vi "Dashboard Main.vi"() -> ()   [LabVIEW 2017]
uses:
  <vilib>/Utility/miscctls.llb/LVRowAndColumnTypeDef.ctl
  <vilib>/event_ctls.llb/eventvkey.ctl
  <vilib>/Rock Robotics/Network Tables/NT Read Numeric Array.vi
  <vilib>/Rock Robotics/Network Tables/NT Read Boolean.vi
  <vilib>/Rock Robotics/Network Tables/NT Write Boolean.vi
  <vilib>/Rock Robotics/WPI/Dashboard/WPI_DashboardLogging Global.vi
panel:
  in  "Camera Settings Right":T1={"Frame Rate"=30, "Compression"=30, "Size"=1, "DB Camera Config"=FALSE} {"Frame Rate" scale=1.0..30.0; "Compression" scale=100.0..-1.0; "Size" items=["640x480", "320x240", "160x120"]}
  in  "Camera Name Right":string(combo)="No Camera Selection"
  out "Camera Info":cluster{"Mbps LED":bool, "Mbps":dbl, "fps":dbl} {"fps" format="%#.1g"; "Mbps" format="%#.1g"}
  in  "Camera Settings":T1={"Frame Rate"=30, "Compression"=30, "Size"=1, "DB Camera Config"=FALSE} {"Frame Rate" scale=1.0..30.0; "Compression" scale=100.0..-1.0; "Size" items=["640x480", "320x240", "160x120"]}
  in  "TCP":refnum<k5>
  in  "Rec Mode":enum32{"Stop", "Record", "Playback"}(radio)
  out "Robot IP":string
  out "Image Message":string="Timeout in Camera Communications"
  in  "Dashboard Tab":T2(tab)
  in  "Select Auto":string(combo)="Select Autonomous ..."
  out "NT Connection":bool
  out "MotorChart R":cluster{"Numeric":dbl, "Numeric":dbl}(graph)
  out "MotorChart L":cluster{"Numeric":dbl, "Numeric":dbl}(graph)
  out "MotorSliders R":cluster{"MotorSlide1":dbl, "MotorSlide2":dbl} {"MotorSlide2" scale=-1.0..1.0 scale format="%#_2e"; "MotorSlide1" scale=-1.0..1.0 scale format="%#_2e"}
  out "MotorSliders L":cluster{"MotorSlide1":dbl, "MotorSlide2":dbl} {"MotorSlide2" scale=-1.0..1.0 scale format="%#_2e"; "MotorSlide1" scale=-1.0..1.0 scale format="%#_2e"}
  out "JS1 Z":dbl(slide) scale=-1.0..1.0 scale format="%#_2e"
  out "JS1 Graph":cluster{"X":dbl, "Y":dbl}[](graph)
  out "JS1 Buttons":T3
  out "JS2 Z":dbl(slide) scale=-1.0..1.0 scale format="%#_2e"
  out "JS2 Graph":cluster{"X":dbl, "Y":dbl}[](graph)
  out "JS2 Buttons":T3
  out "Mode":T4(ring)=enum."Auto Disabled"
  out "Camera Image Right":T5(plugin-control)
  in  "Go Fast":bool
  in  "Trim":dbl(slide) scale=0.0..1.0
  in  "Forward?":bool
  in  "If you want to go straight, how far?":dbl
  in  "How fast do you want it to go?":dbl
  in  "If you want to deliver a cube, where?":string(combo)
  in  "Which Auto Program do you want?":string(combo)
  out "Upper lift limit":bool
  out "lower lift limit":bool
  out "gyro":dbl(knob) scale=0.0..360.0
  out "Gauge":dbl(knob) scale=0.0..90.0
  in  "Clear Sticky Faults":bool
  in  "Intake Angle Speed":dbl
  out "Intake angle encoder":dbl
  out "NavX Pitch":dbl
  out "Right encoder":dbl
  out "Pigeon Pitch":dbl
  out "left encoder":dbl
  in  "Test Slider":dbl(slide) scale=0.0..100.0 scale format="%#_3g"
  in  "On/Off":bool caption="Solenoid"
  in  "Test Name":u16(ring) items=["Select the test to run..."]
  in  "Test Tree":string(tree)
  in  "Motor":cluster{"Value":dbl, "Enable":bool} {"Value" scale=-1.0..1.0 scale format="%#_3g"}
  out "Progress":T6 {"Test Progress" scale=0.0..100.0}
  in  "Rev/Fwd":cluster{"Forward":bool, "Reverse":bool}
  in  "Test Ring":u16(ring) items=["Monochrome", "Color"]
  out "Cmd Status":string
  in  "Execute Command":bool
  in  "Command Params":string[][](table)
  in  "Command Selection":i32(listbox)
  in  "CheckList":i32(listbox)
  out "Tree":string(tree)
  out "Camera Image":T5(plugin-control)
  out "Background":bool
  in  "Camera Name":string(combo)="No Camera Selection"
  # "HW"
  # "HW"
  # "Joysticks"
  # "Drive Motors"
  # "Front"
  # "Right"
  # "Left"
  # "Back"
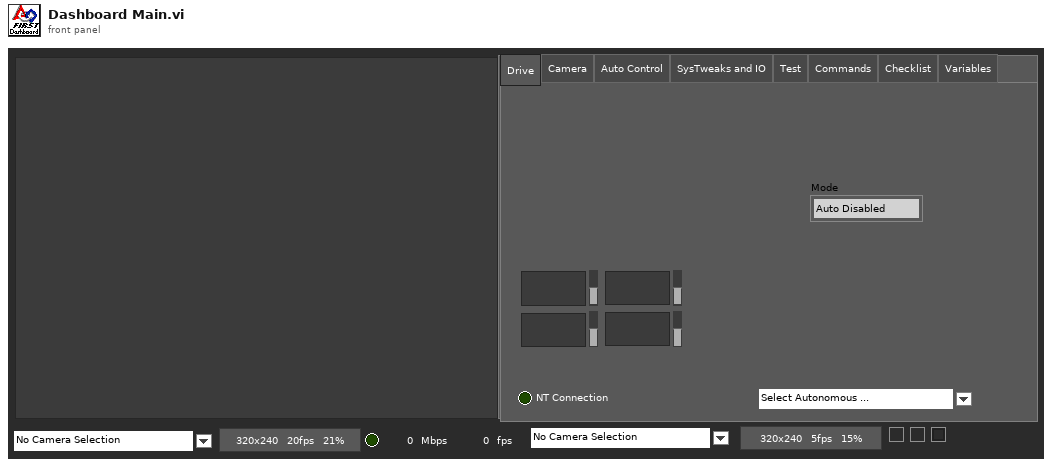
[diagram p1: front panel]
types:
  T1 = cluster{"Frame Rate":i32, "Compression":i32, "Size":u16, "DB Camera Config":bool}
  T2 = enum32{"Drive", "Camera", "Auto Control", "SysTweaks and IO", "Test", "Commands", "Checklist", "Variables"}
  T3 = cluster{bool, bool, bool, bool, bool, bool, bool, bool, bool, bool, bool, bool}
  T4 = enum8{"Tele-Op Disabled", "Tele-Op Enabled", "Auto Disabled", "Auto Enabled", "Test Disabled", "Test Enabled", "Disconnected", "No Code", "E-Stop"}
  T5 = typedef "IMAQ Image.ctl" = refnum<image>
  T6 = cluster{"Test Progress":u8, "Test Progress Text":string}
  T7 = cluster{"Save Path":path, "Interval (s)":dbl, "Keep":i32}
  T8 = enum32{"Drive", "Camera", "Basic", "Custom", "Test", "Commands", "Checklist", "Variables"}
  T9 = typedef "Image Type" = u32
  T10 = cluster{"IDs":cluster{"RPC field ID":u16, "Unique ID":u16}, "String":string}
  T11 = cluster{"Error Strings":string, "Disable Counts":cluster{u16, u16}, "Rail Faults":cluster{u16, u16, u16}, "Robot IP":string, "DB Mode":u8, "Event Info":cluster{"Name":string, "Type":u8, "Number":u16, "Replay":u8}}
  T12 = cluster{"Storage":cluster{"Disk Free":u64, "RAM Block":u32, "RAM free":u32}, "CPU Utilization":cluster{"CPU % ISR":sgl, "CPU % Time Crit":sgl, "CPU % Timed Str":sgl, "CPU % High":sgl, "CPU % Above":sgl, "CPU % Normal":sgl, "CPU % Low":sgl}, "CAN":cluster{"% Bus Utilization":sgl, "Bus Off Cnt":u32, "TX_FIFO Full Cnt":u32, "Receive Error Cnt":u8, "Transmit Error Cnt":u8}, "HID":cluster{"HID Outputs":u32, "Rumble Low":u16, "Rumble High":u16}[]}
  T13 = cluster{"Status bits":cluster{"Test Mode":bool, "Autonomous":bool, "Enabled":bool, "Code Start":bool, "Brownout":bool, "Reserved 2":bool, "Reserved 3":bool, "E-Stop":bool}, "Code Trace":cluster{"Disabled":bool, "TeleOp":bool, "Auto":bool, "Test":bool}, "Controller Type":enum16{"unknown", "cRIO", "roboRio"}, "Code?":enum16{"unknown", "noCode", "code"}, "Battery V":dbl}
  T14 = cluster{"Control Bits":cluster{"TestMode":bool, "Autonomous":bool, "Enabled":bool, "FMS Present":bool, bool, bool, bool, "E-Stop":bool}, "Team Station ":u8, "Countdown":sgl, "Joystick Values":cluster{"Axes":dbl[], "Buttons":bool[], "POVs":i16[]}[]}
  T15 = cluster{"Axes":dbl[], "Buttons":bool[], "POVs":i16[]}[]
  T16 = cluster{"Numeric Array[0]":dbl, "Numeric Array[1]":dbl, "Numeric Array[2]":dbl, "Numeric Array[3]":dbl, "Numeric Array[4]":dbl, "Numeric Array[5]":dbl, "Numeric Array[6]":dbl, "Numeric Array[7]":dbl, "Numeric Array[8]":dbl}
  T17 = cluster{"Axes":dbl[], "Buttons":bool[], "POVs":i16[]}
  T18 = cluster{"Buttons[0]":bool, "Buttons[1]":bool, "Buttons[2]":bool, "Buttons[3]":bool, "Buttons[4]":bool, "Buttons[5]":bool, "Buttons[6]":bool, "Buttons[7]":bool, "Buttons[8]":bool, "Buttons[9]":bool, "Buttons[10]":bool, "Buttons[11]":bool}
  T19 = cluster{"Camera Image":refnum<vi>, "Dashboard Tab":refnum<vi>, "Background":refnum<vi>, "Rec Mode":refnum<vi>, "Test Slider":refnum<vi>, "On/Off ":refnum<vi>, "Test Ring":refnum<vi>, "Rev/Fwd":refnum<vi>, "Test Name":refnum<vi>, "Motor":refnum<vi>, "Progress":refnum<vi>, "CheckList":refnum<vi>, "Tree":refnum<vi>, "Test Tree":refnum<vi>, "Command Params":refnum<vi>, "Command Selection":refnum<vi>, "Execute Command":refnum<vi>, "Cmd Status":refnum<vi>, "Camera Settings":refnum<vi>, "Camera Name":refnum<vi>, "Camera Info":refnum<vi>, "Camera Settings Right":refnum<vi>, "Camera Name Right":refnum<vi>, "Camera Image Right":refnum<vi>}
  T20 = cluster{"Camera Name Right":string, string, "Saved DB Images Info":cluster{"Save Path":path, "Interval (s)":dbl, "Keep":i32}}
  T21 = cluster{"Camera Name":string, string, "Saved DB Images Info":cluster{"Save Path":path, "Interval (s)":dbl, "Keep":i32}}
  T22 = cluster{"Operation":enum16{"Update", "Clear"}, "Color Box":u32}[]
  T23 = typedef "eventvkey.ctl" = enum16{"ASCII", "Enter", "Return", "Shift", "Ctrl", "Alt", "Cmd", "Opt", "Caps", "NumLock", "Clear", "Break", "Up", "Down", "Left", "Right", "Insert", "Delete", "Home", "End", "PageUp", "PageDown", "Escape", "Help", "Pause", "ScrollLock", "F1", "F2", "F3", "F4", "F5", "F6", "F7", "F8", "F9", "F10", "F11", "F12", "F13", "F14", "F15", "F16", "F17", "F18", "F19", "F20", "F21", "F22", "F23", "F24", "Play", "VolumeUp", "VolumeDown", "Mute", "Two Byte Char"}
  T24 = cluster{"Image Size":bool, "Image Type":bool, "Pixel Value":bool, "ROI Information":bool, "Zoom Factor":bool}
  T25 = cluster{"Operation":enum16{"Update", "Clear"}, "Color Box":u32}
  T26 = typedef "LVRowAndColumnTypeDef.ctl" = cluster{"Row":i32, "Column":i32}
  T27 = cluster{"Shift":bool, "Ctrl":bool, "Alt":bool, "Cmd":bool, "Opt":bool}
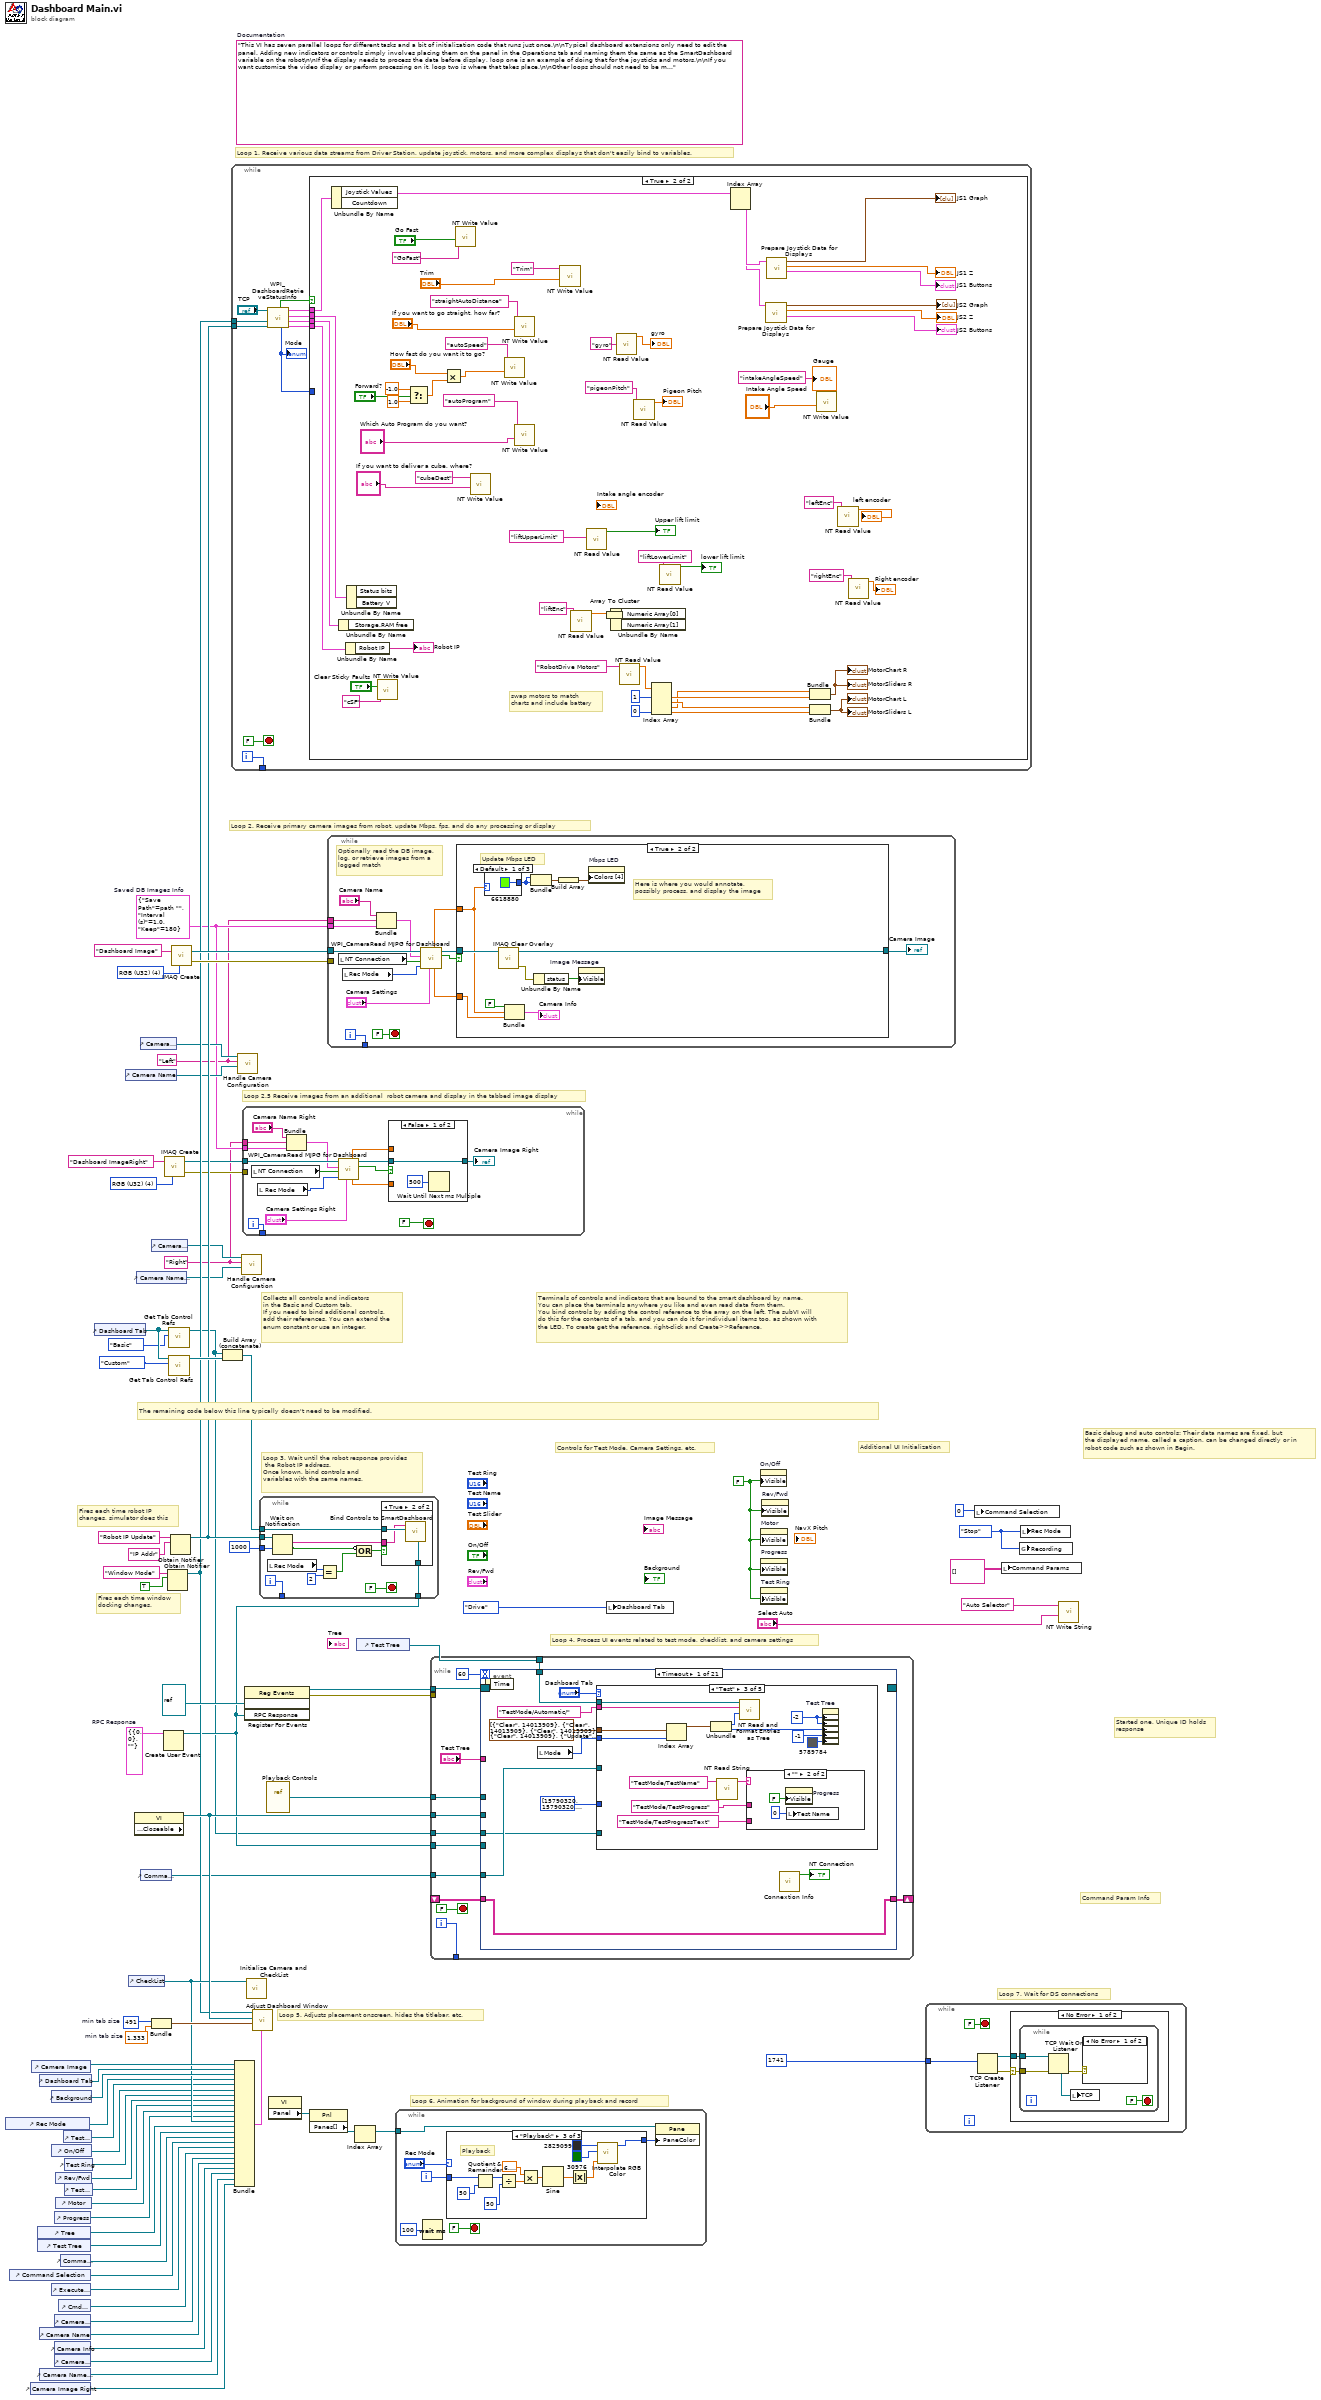
[diagram p0: block diagram]
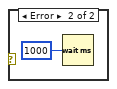
[diagram p3: hidden frame]
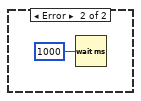
[diagram p4: hidden frame]
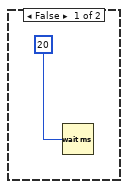
[diagram p5: hidden frame]
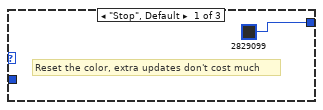
[diagram p6: hidden frame]
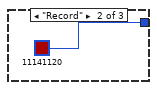
[diagram p7: hidden frame]
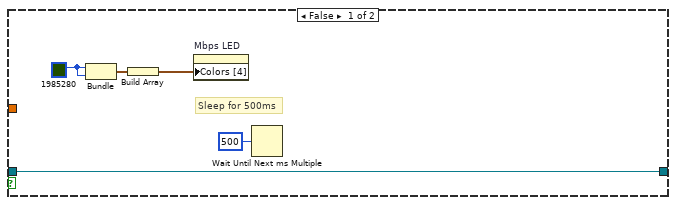
[diagram p9: hidden frame]
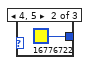
[diagram p10: hidden frame]
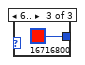
[diagram p11: hidden frame]
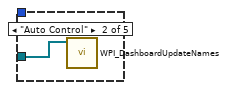
[diagram p13: hidden frame]
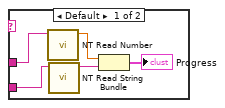
[diagram p14: hidden frame]
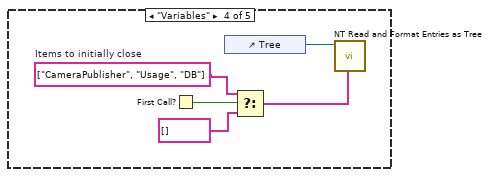
[diagram p15: hidden frame]
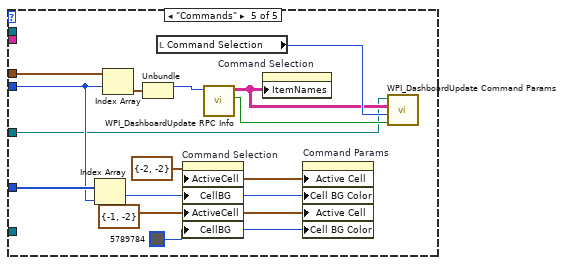
[diagram p16: hidden frame]
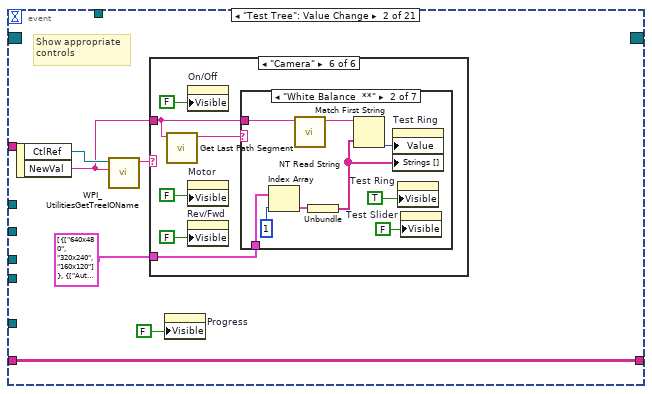
[diagram p17: hidden frame]
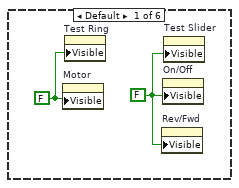
[diagram p18: hidden frame]
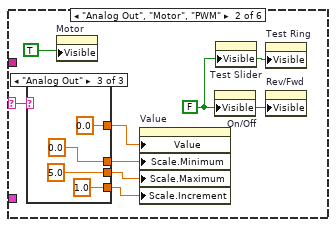
[diagram p19: hidden frame]
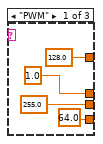
[diagram p20: hidden frame]
diagram:
  w3 = T7 {"Save Path"=path "", "Interval (s)"=1.0, "Keep"=180}  # Saved DB Images Info
  w2 = "Right"
  w1 = "Left"
  w13 = T9 4 items=["Grayscale (U8)", "Grayscale (I16)", "Grayscale (SGL)", "Complex (CSG)", "RGB (U32)", "HSL (U32)", "RGB (U64)"] ("Image Type")
  w29 = T10 {"IDs"={"RPC field ID"=0, "Unique ID"=0}, "String"=""}  # RPC Response
  w52 = 491  # min tab size
  w51 = 1.333  # min tab size
  w59 = enum32{"Stop", "Record", "Playback"}."Stop" ("Rec Mode")
  w36 = FALSE ("Visible")
  (unwired) "This VI has seven parallel loops for different tasks and a bit of initialization code that runs just once.\n\nTypical dashboard extensions only need to edit the panel. Adding new indicators or controls simply involves placing them on the panel in the Operations tab and naming them the same as the SmartDashboard variable on the robot\n\nIf the display needs to process the data before display, loop one is an example of doing that for the joysticks and motors.\n\nIf you want customize the video display or perform processing on it, loop two is where that takes place.\n\nOther loops should not need to be modified. They are pretty standard, and document the task they perform."  # Documentation
  w76 = T9 4 items=["Grayscale (U8)", "Grayscale (I16)", "Grayscale (SGL)", "Complex (CSG)", "RGB (U32)", "HSL (U32)", "RGB (U64)"] ("Image Type")
  # "Loop 2.5 Receive images from an additional  robot camera and display in the tabbed image display"
  # "Command Param Info"
  # "Started one, Unique ID holds\nresponse"
  # "Loop 7. Wait for DS connections"
  # "Basic debug and auto controls: Their data names are fixed, but\nthe displayed name, called a caption, can be changed directly or in\nrobot code such as shown in Begin."
  # "Controls for Test Mode, Camera Settings, etc."
  # "Additional UI Initialization"
  # "Loop 6. Animation for background of window during playback and record"
  # "Fires each time robot IP\nchanges, simulator does this"
  # "Fires each time window\ndocking changes."
  # "Collects all controls and indicators\nin the Basic and Custom tab.\nIf you need to bind additional controls,\nadd their references. You can extend the\nenum constant or use an integer."
  # "The remaining code below this line typically doesn't need to be modified."
  # "Loop 4. Process UI events related to test mode, checklist, and camera settings"
  # "Terminals of controls and indicators that are bound to the smart dashboard by name.\nYou can place the terminals anywhere you like and even read data from them.\nYou bind controls by adding the control reference to the array on the left. The subVI will\ndo this for the contents of a tab, and you can do it for individual items too, as shown with\nthe LED. To create get the reference, right-click and Create>>Reference."
  # "Loop 3. Wait until the robot response provides\n the Robot IP address.\nOnce known, bind controls and\nvariables with the same names."
  # "Loop 5. Adjusts placement onscreen, hides the titlebar, etc."
  # "Loop 1. Receive various data streams from Driver Station, update joystick, motors, and more complex displays that don't easily bind to variables."
  # "Loop 2. Receive primary camera images from robot, update Mbps, fps, and do any processing or display"
  n1 = control-ref of="Rec Mode"() -> (w42:refnum<vi>)
  n2 = control-ref of="Command Selection"() -> (w28:refnum<vi>)
  n3 = control-ref of="Camera Image Right"() -> (w6:refnum<vi>)
  n4 = control-ref of="Camera Image"() -> (w54:refnum<vi>)
  n5 = control-ref of="Tree"() -> (w46:refnum<vi>)
  n6 = control-ref of="Test Tree"() -> (w45:refnum<vi>)
  n7 = control-ref of="Dashboard Tab"() -> (w53:refnum<vi>)
  n8 = control-ref of="Camera Name"() -> (w19:refnum<vi>)
  n9 = control-ref of="Camera Name Right"() -> (w7:refnum<vi>)
  n10 = control-ref of="Execute Command"() -> (w30:refnum<vi>)
  n11 = control-ref of="Background"() -> (w49:refnum<vi>)
  n12 = control-ref of="On/Off"() -> (w40:refnum<vi>)
  n13 = control-ref of="Progress"() -> (w37:refnum<vi>)
  n14 = control-ref of="Camera Settings"() -> (w20:refnum<vi>)
  n15 = control-ref of="Camera Info"() -> (w18:refnum<vi>)
  n16 = control-ref of="Camera Settings Right"() -> (w8:refnum<vi>)
  n17 = control-ref of="Rev/Fwd"() -> (w38:refnum<vi>)
  n18 = control-ref of="Motor"() -> (w43:refnum<vi>)
  n19 = control-ref of="Cmd Status"() -> (w24:refnum<vi>)
  n20 = control-ref of="Command Params"() -> (w31:refnum<vi>)
  n21 = control-ref of="Test Slider"() -> (w41:refnum<vi>)
  n22 = control-ref of="Test Ring"() -> (w39:refnum<vi>)
  n23 = control-ref of="Test Name"() -> (w44:refnum<vi>)
  n24 = control-ref of="Dashboard Tab"() -> (w57:refnum<vi>)
  n25 = control-ref of="Camera Name"() -> (w21:refnum<vi>)
  n26 = control-ref of="CheckList"() -> (w47:refnum<vi>)
  n27 = property class="VI" props=["Front Panel.Closeable"]() -> (reference out=w58:refnum<vi>)  [unwired: 2 in, 2 out]
  n28 = control-ref of="Camera Name Right"() -> (w9:refnum<vi>)
  n29 = control-ref of="Camera Settings"() -> (w22:refnum<vi>)
  n30 = control-ref of="Command Params"() -> (w23:refnum<vi>)
  n31 = control-ref of="Camera Settings Right"() -> (w10:refnum<vi>)
  n32 = Bundle("min tab size"=w52, "min tab size"=w51) -> (w50:cluster{"min tab size":i32, "min tab size":dbl})  [unwired: 1 in]
  n33 = Create User Event(user event datatype=w29) -> (user event=w25:refnum<user-event>)  [unwired: 1 in, 1 out]
  n34 = call "IMAQ Create"("Image Name"="Dashboard ImageRight", "Image Type"=w13) -> ("New Image"=w12:T5, "error out"=w11:errorcluster)  [unwired: 2 in, 1 out]
  n35 = Obtain Notifier(name (unnamed)="Window Mode", notification data type=TRUE) -> (notifier out=w34:refnum<notifier>)  [unwired: 2 in, 2 out]
  n36 = call <vilib>:"Get Tab Control Refs.vi"("Page Index"=T8."Basic" ("Dashboard Tab"), "TabControl in"=w57) -> ("ControlsOnPage"=w17:refnum<vi>[])  [unwired: 9 in]
  n37 = call <vilib>:"Get Tab Control Refs.vi"("Page Index"=T8."Custom" ("Dashboard Tab"), "TabControl in"=w57) -> ("ControlsOnPage"=w56:refnum<vi>[])  [unwired: 9 in]
  n38 = Obtain Notifier(name (unnamed)="Robot IP Update", notification data type="IP Addr" ("name (unnamed)")) -> (notifier out=w35:refnum<notifier>)  [unwired: 2 in, 2 out]
  n39 = call "IMAQ Create"("Image Name"="Dashboard Image", "Image Type"=w76) -> ("New Image"=w74:T5, "error out"=w73:errorcluster)  [unwired: 2 in, 1 out]
  n40 = Build Array (concatenate)(w17, w56) -> (w55:refnum<vi>[])
  n41 = while {
    tunnel: [w86] -> _
    tunnel: w35 -> [w80]
    tunnel: w34 -> [w77]
    i -> [w86]
    stop <- FALSE stop-if-true
    n42 = call <vilib>:"WPI_DashboardRetrieveStatusInfo.vi"("Binding Refnum"=w80, "Window Mode Notifier"=w77, "TCP Cnx"="TCP") -> ("Power and Errors"=w81:T11, "Robot Metrics"=w84:T12, "Status Info"=w85:T13, "Control Info"=w82:T14, "Robot Mode"=w79:T4, "Process?"=w83:bool)  [unwired: 3 in]
    "Mode" <- w79
    n43 = case shown="True" w83 {
      tunnel: w85 -> [_ w148]
      tunnel: w84 -> [_ w147]
      tunnel: w82 -> [_ w146]
      tunnel: w81 -> [_ w145]
      tunnel: w79 -> [_ _]
      frame False {
        n44 = Wait (ms)(milliseconds to wait=u32 20) -> ()  [unwired: 1 out]
      }
      frame True {
        # "swap motors to match\ncharts and include battery"
        n45 = Unbundle By Name(w146) -> ("Joystick Values"=w136:T15)  [unwired: 1 out]
        n46 = Unbundle By Name(w147) -> ()  [unwired: 1 out]
        n47 = Unbundle By Name(w145) -> ("Robot IP"=→"Robot IP":string)
        n48 = Unbundle By Name(w148) -> ()  [unwired: 2 out]
        n49 = call-poly <vilib>:"NT Write Value.vi"("Boolean"="Clear Sticky Faults", "Name"="cSF") -> ()  [unwired: 9 in, 1 out]
        n50 = Select(t=-1.0, s="Forward?", f=1.0) -> (s? t:f=w93:dbl)
        n51 = Multiply(x="How fast do you want it to go?", y=w93) -> (x*y=w95:dbl)
        n52 = call-poly <vilib>:"NT Write Value.vi"("Boolean"="Go Fast", "Name"="GoFast") -> ()  [unwired: 9 in, 1 out]
        n53 = call-poly <vilib>:"NT Write Value.vi"("String"="If you want to deliver a cube, where?", "Name"="cubeDest") -> ()  [unwired: 9 in, 1 out]
        n54 = call-poly <vilib>:"NT Write Value.vi"("Numeric"=w95, "Name"="autoSpeed") -> ()  [unwired: 9 in, 1 out]
        n55 = call-poly <vilib>:"NT Write Value.vi"("Numeric"="If you want to go straight, how far?", "Name"="straightAutoDistance") -> ()  [unwired: 9 in, 1 out]
        n56 = call-poly <vilib>:"NT Write Value.vi"("String"="Which Auto Program do you want?", "Name"="autoProgram") -> ()  [unwired: 9 in, 1 out]
        n57 = call-poly <vilib>:"NT Write Value.vi"("Numeric"="Trim", "Name"="Trim") -> ()  [unwired: 9 in, 1 out]
        n58 = call-poly <vilib>:"NT Read Value.vi"("Name"="liftEnc") -> ("Numeric Array"=w90:dbl[])  [unwired: 9 in, 1 out]
        n59 = call-poly <vilib>:"NT Read Value.vi"("Name"="liftUpperLimit") -> ("Boolean"=→"Upper lift limit":bool)  [unwired: 9 in, 1 out]
        n60 = Array To Cluster(array=w90) -> (cluster=w89:T16)
        n61 = Unbundle By Name(w89) -> ()  [unwired: 2 out]
        n62 = call-poly <vilib>:"NT Read Value.vi"("Name"="gyro") -> ("Numeric"=→"gyro":dbl)  [unwired: 9 in, 1 out]
        n63 = call-poly <vilib>:"NT Read Value.vi"("Name"="RobotDrive Motors") -> ("Numeric Array"=w126:dbl[])  [unwired: 9 in, 1 out]
        n64 = call-poly <vilib>:"NT Read Value.vi"("Name"="pigeonPitch") -> ("Numeric"=→"Pigeon Pitch":dbl)  [unwired: 9 in, 1 out]
        n65 = Index Array(array=w126, index #1=1, index #4=0) -> (element #1=w140:dbl, element #2=w141:dbl, element #3=w139:dbl, element #4=w144:dbl)  [unwired: 2 in]
        n66 = call-poly <vilib>:"NT Read Value.vi"("Name"="liftLowerLimit") -> ("Boolean"=→"lower lift limit":bool)  [unwired: 9 in, 1 out]
        n67 = Index Array(array=w136) -> (element #1=w135:T17, element #2=w131:T17)  [unwired: 2 in]
        n68 = call "Prepare Joystick Data for Displays.vi"("Joystick Values"=w131) -> ("Buttons"=→"JS2 Buttons":T18, "Z Axis"=→"JS2 Z":dbl, "Cartesian Data"=→"JS2 Graph":cluster{"X axis":dbl, "X axis":dbl}[])  [unwired: 8 in]
        n69 = call "Prepare Joystick Data for Displays.vi"("Joystick Values"=w135) -> ("Buttons"=→"JS1 Buttons":T18, "Z Axis"=→"JS1 Z":dbl, "Cartesian Data"=→"JS1 Graph":cluster{"X axis":dbl, "X axis":dbl}[])  [unwired: 8 in]
        n70 = Bundle("Numeric"=w139, "Numeric"=w140) -> (→"MotorChart R" →"MotorSliders R":cluster{"Numeric":dbl, "Numeric":dbl})  [unwired: 1 in]
        n71 = Bundle("Numeric"=w141, "Numeric"=w144) -> (→"MotorChart L" →"MotorSliders L":cluster{"Numeric":dbl, "Numeric":dbl})  [unwired: 1 in]
        n72 = call-poly <vilib>:"NT Write Value.vi"("Numeric"="Intake Angle Speed", "Name"="intakeAngleSpeed") -> ()  [unwired: 9 in, 1 out]
        n73 = call-poly <vilib>:"NT Read Value.vi"("Name"="leftEnc") -> ("Numeric"=→"left encoder":dbl)  [unwired: 9 in, 1 out]
        n74 = call-poly <vilib>:"NT Read Value.vi"("Name"="rightEnc") -> ("Numeric"=→"Right encoder":dbl)  [unwired: 9 in, 1 out]
      }
    }
  }
  n75 = Bundle("Camera Image"=w54, "Dashboard Tab"=w53, "Background"=w49, "Rec Mode"=w42, "Test Slider"=w41, "On/Off"=w40, "Test Ring"=w39, "Rev/Fwd"=w38, "Test Name"=w44, "Motor"=w43, "Progress"=w37, "CheckList"=w47, "Tree"=w46, "Test Tree"=w45, "Command Params"=w31, "Command Selection"=w28, "Execute Command"=w30, "Cmd Status"=w24, "Camera Settings"=w20, "Camera Name"=w19, "Camera Info"=w18, "Camera Settings Right"=w8, "Camera Name Right"=w7, "Camera Image Right"=w6) -> (w48:T19)  [unwired: 1 in]
  n76 = call "Handle Camera Configuration.vi"("CameraNameRef"=w21, "Display Name"=w1, "ClusterRef"=w22) -> ()  [unwired: 9 in]
  n77 = call "Handle Camera Configuration.vi"("CameraNameRef"=w9, "Display Name"=w2, "ClusterRef"=w10) -> ()  [unwired: 9 in]
  n78 = while {
    tunnel: w12 -> [w163]
    tunnel: w11 -> [_]
    tunnel: [w158] -> _
    tunnel: w3 -> [w152]
    tunnel: w2 -> [w149]
    i -> [w158]
    stop <- FALSE stop-if-true
    n79 = local read "NT Connection"() -> (w153:bool)
    n80 = local read "Rec Mode"() -> (w162:enum32{"Stop", "Record", "Playback"})
    n81 = Bundle("Camera Name Right"="Camera Name Right", w149, "Saved DB Images Info"=w152) -> (w151:T20)  [unwired: 1 in]
    n82 = call <vilib>:"WPI_CameraRead MJPG for Dashboard.vi"("Camera Settings"="Camera Settings Right", "Rec Mode"=w162, "NT Connection"=w153, "Capture Info"=w151, "Refnum in"=w163) -> ("Active"=w157:bool, "Refnum out"=w160:T5, "FPS"=w155:dbl, "Bandwidth (Mbps)"=w156:dbl)  [unwired: 3 in]
    n83 = case shown="False" w157 {
      tunnel: w160 -> [w164 w166]
      tunnel: w156 -> [_ _]
      tunnel: w155 -> [_ _]
      tunnel: [w164 w166] -> w154
      frame False {
        n84 = Wait Until Next ms Multiple(millisecond multiple=u32 500) -> ()  [unwired: 1 out]
      }
      frame True {
      }
    }
    "Camera Image Right" <- w154
  }
  n85 = register-events(refnum<vi> refnum, w25) -> (reference out=w63:refnum<event-registration>, error out=w62:errorcluster)  [unwired: 2 in]
  n86 = call "Initialize Camera and CheckList.vi"("ListBox in"=w47) -> ()  [unwired: 11 in]
  n87 = call "Adjust Dashboard Window.vi"("Sizing Refnums"=w48, "Size Constraints"=w50, "VI"=w58, "WIn Mode"=w34) -> ()  [unwired: 8 in]
  n88 = while {
    tunnel: w55 -> [w178]
    tunnel: w35 -> [w176]
    tunnel: [w174] -> _
    tunnel: u32 1000 ("milliseconds to wait") -> [w173]
    tunnel: w25 -> [w167]
    i -> [w174]
    stop <- FALSE stop-if-true
    n89 = local read "Rec Mode"() -> (w169:enum32{"Stop", "Record", "Playback"})
    n90 = Wait on Notification(notifier=w176, timeout in ms (-1)=w173) -> (notification=w175:string, timed out?=w171:bool)  [unwired: 2 in, 2 out]
    n91 = Equal?(x=w169, y=u16 2 ("Rec Mode")) -> (x = y?=w170:bool)
    n92 = Compound Arithmetic op=OR(invert w171, w170) -> (w172:bool)
    n93 = case shown="True" w172 {
      tunnel: w178 -> [_ w181]
      tunnel: w175 -> [_ w180]
      tunnel: w167 -> [_ w179]
      frame False {
      }
      frame True {
        n94 = call <vilib>:"Bind Controls to SmartDashboard.vi"("RPC ref"=w179, "Bound Control Refs"=w181, "Server IP Address"=w180) -> ()  [unwired: 9 in]
      }
    }
  }
  n95 = vi-ref "Playback Controls.vi"() -> (w64:refnum<vi>)
  n96 = property class="VI"() -> ("Panel"=w66:refnum<vi>)  [unwired: 2 in, 2 out]
  n97 = property class="Pnl"(reference=w66) -> ("Panes[]"=w67:refnum<vi>[])  [unwired: 1 in, 2 out]
  n98 = while {
    tunnel: w74 -> [w194]
    tunnel: w73 -> [_]
    tunnel: [w195] -> _
    tunnel: w3 -> [w185]
    tunnel: w1 -> [w182]
    i -> [w195]
    stop <- FALSE stop-if-true
    # "Optionally read the DB image,\nlog, or retrieve images from a\nlogged match"
    n99 = local read "NT Connection"() -> (w186:bool)
    n100 = local read "Rec Mode"() -> (w190:enum32{"Stop", "Record", "Playback"})
    n101 = Bundle("Camera Name"="Camera Name", w182, "Saved DB Images Info"=w185) -> (w184:T21)  [unwired: 1 in]
    n102 = call <vilib>:"WPI_CameraRead MJPG for Dashboard.vi"("Camera Settings"="Camera Settings", "Rec Mode"=w190, "NT Connection"=w186, "Capture Info"=w184, "Refnum in"=w194) -> ("Active"=w192:bool, "Refnum out"=w193:T5, "FPS"=w191:dbl, "Bandwidth (Mbps)"=w189:dbl)  [unwired: 3 in]
    n103 = case shown="True" w192 {
      tunnel: w193 -> [w197 w208]
      tunnel: w189 -> [_ w205]
      tunnel: w191 -> [_ w206]
      tunnel: [w197 w202] -> w187
      frame False {
        w199 = u32 1985280 ("Color Box")
        # "Sleep for 500ms"
        n104 = Bundle("Color Box"=w199, "Color Box"=w199) -> (w200:cluster{"Color Box":u32, "Color Box":u32})  [unwired: 1 out]
        n105 = Build Array(w200) -> (w198:cluster{"Color Box":u32, "Color Box":u32}[])
        n106 = property on="Mbps LED" class="Bool (strict)"("Colors [4]"=w198) -> ()  [unwired: 2 in, 2 out]
        n107 = Wait Until Next ms Multiple(millisecond multiple=u32 500) -> ()  [unwired: 1 out]
      }
      frame True {
        # "Here is where you would annotate,\npossibly process, and display the image"
        # "Update Mbps LED"
        n108 = case shown="Default" w205 {
          tunnel: [u32 6618880 ("Color Box") u32 16776722 ("Color Box") u32 16716800 ("Color Box")] -> w209
          frame Default {
          }
          frame 4, 5 {
          }
          frame 6.. {
          }
        }
        n109 = call "IMAQ Clear Overlay"("Image"=w208) -> ("error out"=w211:errorcluster, "Image Out"=w202:T5)  [unwired: 2 in, 7 out]
        n110 = Bundle(FALSE, "Bandwidth (Mbps)"=w205, "FPS"=w206) -> (→"Camera Info":cluster{bool, "Bandwidth (Mbps)":dbl, "FPS":dbl})  [unwired: 1 in]
        n111 = Bundle("Color Box"=w209, "Color Box"=w209) -> (w210:cluster{"Color Box":u32, "Color Box":u32})  [unwired: 1 out]
        n112 = Unbundle By Name(w211) -> ("status"=w212:bool)
        n113 = Build Array(w210) -> (w207:cluster{"Color Box":u32, "Color Box":u32}[])
        n114 = property on="Image Message" class="Str"("Visible"=w212) -> ()  [unwired: 2 in, 2 out]
        n115 = property on="Mbps LED" class="Bool (strict)"("Colors [4]"=w207) -> ()  [unwired: 2 in, 2 out]
      }
    }
    "Camera Image" <- w187
  }
  n116 = Index Array(array=w67) -> (element=w65:refnum<vi>)  [unwired: 1 in]
  n117 = control-ref of="Test Tree"() -> (w68:refnum<vi>)
  n118 = while {
    tunnel: w65 -> [w217]
    i -> [w220]
    stop <- FALSE stop-if-true
    n119 = Wait (ms)(milliseconds to wait=u32 100) -> ()  [unwired: 1 out]
    n120 = case shown="\"Playback\"" "Rec Mode" {
      tunnel: w220 -> [_ _ w235]
      tunnel: [u32 2829099 ("Base Color") u32 11141120 ("Target Color") w224] -> w216
      frame "Stop", Default {
        # "Reset the color, extra updates don't cost much"
      }
      frame "Record" {
      }
      frame "Playback" {
        # "Playback"
        n121 = Quotient & Remainder(x=w235, y=u32 50 ("milliseconds to wait")) -> (x-y*floor(x/y)=w231:u32)  [unwired: 1 out]
        n122 = Divide(x=w231, y=u32 50 ("milliseconds to wait")) -> (x/y=w228:dbl)
        n123 = Multiply(x=6.283185307179586, y=w228) -> (x*y=w233:dbl)
        n124 = Sine(x=w233) -> (sin(x)=w232:dbl)
        n125 = Absolute Value(x=w232) -> (abs(x)=w225:dbl)
        n126 = call "Interpolate RGB Color.vi"("Proportion"=w225, "Target Color"=u32 30976, "Base Color"=u32 2829099) -> ("Result Color"=w224:u32)  [unwired: 8 in]
      }
    }
    n127 = property class="Pane"(reference=w217, "PaneColor"=w216) -> ()  [unwired: 1 in, 2 out]
  }
  n128 = while {
    tunnel: [w245] -> _
    tunnel: w68 -> [w244]
    tunnel: w64 -> [w243]
    tunnel: w63 -> [w242]
    tunnel: w62 -> [_]
    tunnel: w58 -> [w241]
    tunnel: w25 -> [w240]
    tunnel: w23 -> [w239]
    shift-right: [w238] -> _
    shift-left: _ -> [w237]
    tunnel: w17 -> [w236]
    i -> [w245]
    stop <- FALSE stop-if-true
    n129 = event shown="[0] Timeout" {
      selector: w242 -> [_ _ _ _ _ _ _ _ _ _ _ _ _ _ _ _ _ _ _ _ _]
      dyn-events: [_ _ _ _ _ _ _ _ _ _ _ _ _ _ _ _ w505 _ _ _ _] -> _
      timeout: u32 60 ("milliseconds to wait") -> [_ _ _ _ _ _ _ _ _ _ _ _ _ _ _ _ _ _ _ _ _]
      tunnel: w244 -> [w257 _ _ _ _ _ _ _ _ _ _ _ _ _ _ _ _ _ _ _ _]
      tunnel: "Test Tree" -> [_ _ _ _ _ _ _ _ _ _ _ w472 w480 w482 w486 w494 _ _ _ _ _]
      tunnel: w243 -> [_ _ _ _ _ _ _ _ _ _ _ _ _ _ _ _ w507 _ w525 _ _]
      tunnel: w241 -> [_ _ _ _ _ _ _ _ _ _ _ _ _ _ _ _ w503 _ _ _ _]
      tunnel: w240 -> [_ _ _ _ _ _ _ _ _ _ _ _ _ _ _ _ w501 _ _ _ _]
      tunnel: w239 -> [w252 _ _ _ _ _ w423 _ _ _ _ _ _ _ _ _ _ _ _ _ _]
      tunnel: [w251 w300 w402 w407 w416 w420 w421 w430 w440 w447 w459 w471 w478 w481 w485 w493 w500 w520 w522 w526 w539] -> w238
      tunnel: w237 -> [w251 w300 w402 w407 w416 w420 w421 _ _ w447 w459 w471 w478 w481 w485 w493 w500 w520 w522 w526 w539]
      tunnel: w236 -> [w249 _ _ _ _ _ _ _ _ _ _ _ _ _ _ _ _ _ _ _ _]
      event Timeout {
        n130 = event-data() -> ()  [unwired: 1 in, 1 out]
        n131 = local read "Mode"() -> (w254:T4)
        n132 = case shown="\"Test\"" "Dashboard Tab" {
          tunnel: w257 -> [_ _ w273 _ _]
          tunnel: "TestMode/Automatic/" ("Name Pattern") -> [_ _ w272 _ _]
          tunnel: T22 [{"Operation"=enum."Clear", "Color Box"=14013909}, {"Operation"=enum."Clear", "Color Box"=14013909}, {"Operation"=enum."Clear", "Color Box"=14013909}, {"Operation"=enum."Clear", "Color Box"=14013909}, {"Operation"=enum."Update", "Color Box"=14013909}, {"Operation"=enum."Update", "Color Box"=16777215}, {"Operation"=enum."Clear", "Color Box"=14013909}, {"Operation"=enum."Clear", "Color Box"=14013909}, {"Operation"=enum."Clear", "Color Box"=14013909}] -> [_ _ w265 _ w293]
          tunnel: w254 -> [_ _ w264 _ w292]
          tunnel: u32[] [15790320, 15790320, 15790320, 15790320, 16777215, 16777215, 15790320, 15790320, 15790320] -> [_ _ _ _ w298]
          tunnel: w252 -> [_ _ _ _ w286]
          tunnel: w249 -> [_ w259 _ _ _]
          frame "SysTweaks and IO", Default {
          }
          frame "Auto Control" {
            n133 = call <vilib>:"WPI_DashboardUpdateNames.vi"("Controls on Tab"=w259) -> ()  [unwired: 11 in]
          }
          frame "Test" {
            w271 = -2 ("Active Item:Row Number")
            n134 = Index Array(array=w265, index=w264) -> (element=w266:T25)
            n135 = Unbundle(w266) -> ("Operation"=w267:enum16{"Update", "Clear"}, "Color Box"=w268:u32)
            n136 = call <vilib>:"NT Read String.vi"("Name"="TestMode/TestName") -> ("String"=w262:string)  [unwired: 9 in, 1 out]
            n137 = call <vilib>:"NT Read and Format Entries as Tree.vi"("Operation"=w267, "Name Pattern"=w272, "Tree Refnum"=w273) -> ()  [unwired: 7 in, 2 out]
            n138 = case shown="\"\"" w262 {
              tunnel: "TestMode/TestProgress" ("Name") -> [w275 _]
              tunnel: "TestMode/TestProgressText" ("Name") -> [w274 _]
              frame Default {
                n139 = call <vilib>:"NT Read Number.vi"("Name"=w275) -> ("Numeric"=w276:dbl)  [unwired: 9 in, 1 out]
                n140 = call <vilib>:"NT Read String.vi"("Name"=w274) -> ("String"=w277:string)  [unwired: 9 in, 1 out]
                n141 = Bundle("Numeric"=w276, "String"=w277) -> (→"Progress":cluster{"Numeric":dbl, "String":string})  [unwired: 1 in]
              }
              frame "" {
                n142 = property on="Progress" class="Clust (strict)"("Visible"=FALSE) -> ()  [unwired: 2 in, 2 out]
                n143 = local write "Test Name"(u16 0) -> ()
              }
            }
            n144 = property on="Test Tree" class="Tree (strict)"("Active Item Row Number"=w271, "ActiveColNum"=w271, "CellBG"=w268, "Active Item Row Number"=-1 ("Active Item:Row Number"), "CellBG"=u32 5789784 ("Color Box")) -> ()  [unwired: 2 in, 2 out]
          }
          frame "Variables" {
            w283 = string[] ["CameraPublisher", "Usage", "DB"]  # Items to initially close
            n145 = First Call?() -> (First Call?: T/F=w284:bool)
            n146 = control-ref of="Tree"() -> (w285:refnum<vi>)
            n147 = Select(t=w283, s=w284, f=string[] []) -> (s? t:f=w281:string[])
            n148 = call <vilib>:"NT Read and Format Entries as Tree.vi"("Tags to  Close"=w281, "Tree Refnum"=w285) -> ()  [unwired: 8 in, 2 out]
          }
          frame "Commands" {
            w294 = u32 5789784 ("Color Box")
            w295 = T26 {"Row"=-1, "Column"=-2} ("Active Cell:Active Cell")
            w297 = T26 {"Row"=-2, "Column"=-2} ("Active Cell:Active Cell")
            n149 = Index Array(array=w298, index=w292) -> (element=w296:u32)
            n150 = Index Array(array=w293, index=w292) -> (element=w291:T25)
            n151 = Unbundle(w291) -> ("Operation"=w290:enum16{"Update", "Clear"})  [unwired: 1 out]
            n152 = local read "Command Selection"() -> (w289:i32)
            n153 = property on="Command Selection" class="MCListbox (strict)"("ActiveCell"=w297, "CellBG"=w296, "ActiveCell"=w295, "CellBG"=w294) -> ()  [unwired: 2 in, 2 out]
            n154 = call <vilib>:"WPI_DashboardUpdate RPC Info.vi"("Operation"=w290) -> ("update"=w288:bool, "commands"=w287:string[][])  [unwired: 9 in]
            n155 = property on="Command Selection" class="MCListbox (strict)"("ItemNames"=w287) -> ()  [unwired: 2 in, 2 out]
            n156 = property on="Command Params" class="Tbl (strict)"("Active Cell"=w297, "Cell BG Color"=w296, "Active Cell"=w295, "Cell BG Color"=w294) -> ()  [unwired: 2 in, 2 out]
            n157 = call <vilib>:"WPI_DashboardUpdate Command Params.vi"("Update"=w288, "NewVal"=w289, "Commands"=w287, "Param Tbl"=w286) -> ()  [unwired: 7 in, 1 out]
          }
        }
        n158 = call <vilib>:"Connextion Info.vi"() -> ("Connected"=→"NT Connection":bool)  [unwired: 10 in, 1 out]
      }
      event "Test Tree": Value Change {
        # "Show appropriate\ncontrols"
        n159 = event-data() -> ("CtlRef"=w303:refnum<vi>, "NewVal"=w301:string)  [unwired: 1 in]
        n160 = call <vilib>:"WPI_UtilitiesGetTreeIOName.vi"("NewVal"=w301, "TreeControl in"=w303) -> ("I/O Name"=w304:string)  [unwired: 9 in]
        n161 = case shown="\"Camera\"" w304 {
          selector: w304 -> [_ w311 _ w333 w342 _]
          tunnel: w301 -> [_ _ w330 w332 _ w349]
          tunnel: cluster{string[]}[] [{["640x480", "320x240", "160x120"]}, {["Auto", "Fixed indoor", "Fixed outdoor 1", "Fixed outdoor 2", "Fixed fluorescent 1", "Fixed fluorescent 2", "Hold current"]}, {["Auto", "Flicker-free 50 Hz", "Flicker-free 60 Hz", "Hold current"]}, {["None", "Prioritize frame rate", "Prioritize image quality"]}, {["Monochrome", "Color"]}] -> [_ _ _ _ _ w348]
          frame Default {
            w306 = FALSE ("Visible")
            w305 = FALSE ("Visible")
            n162 = property on="Motor" class="Clust (strict)"("Visible"=w305) -> ()  [unwired: 2 in, 2 out]
            n163 = property on="Test Ring" class="Ring (strict)"("Visible"=w305) -> ()  [unwired: 2 in, 2 out]
            n164 = property on="Rev/Fwd" class="Clust (strict)"("Visible"=w306) -> ()  [unwired: 2 in, 2 out]
            n165 = property on="On/Off" class="Bool (strict)"("Visible"=w306) -> ()  [unwired: 2 in, 2 out]
            n166 = property on="Test Slider" class="Slide (strict)"("Visible"=w306) -> ()  [unwired: 2 in, 2 out]
          }
          frame "Analog Out", "Motor", "PWM" {
            w312 = FALSE ("Visible")
            n167 = case shown="\"Analog Out\"" w311 {
              tunnel: [1.0 ("Value") -1.0 ("Value") 0.0 ("Value")] -> w310
              tunnel: [255.0 ("Value") 1.0 ("Value") 5.0 ("Value")] -> w309
              tunnel: [128.0 ("Value") 0.0 ("Value") 0.0 ("Value")] -> w308
              tunnel: [64.0 ("Value") 0.5 ("Value") 1.0 ("Value")] -> w307
              frame "PWM" {
              }
              frame "Motor", Default {
              }
              frame "Analog Out" {
              }
            }
            n168 = property on="Motor" class="Clust (strict)"("Visible"=TRUE) -> ()  [unwired: 2 in, 2 out]
            n169 = property on="Value" class="Slide (strict)"("Value"=w308, "Scale.Minimum"=w310, "Scale.Maximum"=w309, "Scale.Increment"=w307) -> ()  [unwired: 2 in, 2 out]
            n170 = property on="On/Off" class="Bool (strict)"("Visible"=w312) -> ()  [unwired: 2 in, 2 out]
            n171 = property on="Test Slider" class="Slide (strict)"("Visible"=w312) -> ()  [unwired: 2 in, 2 out]
            n172 = property on="Test Ring" class="Ring (strict)"("Visible"=w312) -> ()  [unwired: 2 in, 2 out]
            n173 = property on="Rev/Fwd" class="Clust (strict)"("Visible"=w312) -> ()  [unwired: 2 in, 2 out]
          }
          frame "Servo" {
            w328 = FALSE ("Visible")
            n174 = call <vilib>:"NT Read Number.vi"("Name"=w330) -> ("Numeric"=w329:dbl)  [unwired: 9 in, 1 out]
            n175 = property on="Test Slider" class="Slide (strict)"("Visible"=TRUE, "Scale.Maximum"=170.0 ("Scale.Range:Maximum")) -> ()  [unwired: 2 in, 2 out]
            n176 = local write "Test Slider"(w329) -> ()
            n177 = property on="Motor" class="Clust (strict)"("Visible"=w328) -> ()  [unwired: 2 in, 2 out]
            n178 = property on="Rev/Fwd" class="Clust (strict)"("Visible"=w328) -> ()  [unwired: 2 in, 2 out]
            n179 = property on="On/Off" class="Bool (strict)"("Visible"=w328) -> ()  [unwired: 2 in, 2 out]
            n180 = property on="Test Ring" class="Ring (strict)"("Visible"=w328) -> ()  [unwired: 2 in, 2 out]
          }
          frame "Relay", "Solenoid" {
            w331 = FALSE ("Visible")
            n181 = property on="Motor" class="Clust (strict)"("Visible"=w331) -> ()  [unwired: 2 in, 2 out]
            n182 = property on="Test Slider" class="Slide (strict)"("Visible"=w331) -> ()  [unwired: 2 in, 2 out]
            n183 = Search and Replace String(input string=w332, search string="/Value  **", replace string="/Direction") -> (result string=w338:string)  [unwired: 5 in, 3 out]
            n184 = property on="Test Ring" class="Ring (strict)"("Visible"=w331) -> ()  [unwired: 2 in, 2 out]
            n185 = call <vilib>:"NT Read String.vi"("Name"=w338) -> ("String"=w336:string)  [unwired: 9 in, 1 out]
            n186 = Equal?(x="Both directions", y=w336) -> (x = y?=w334:bool)
            n187 = Not(x=w334) -> (.not. x?=w335:bool)
            n188 = property on="Rev/Fwd" class="Clust (strict)"("Visible"=w334) -> ()  [unwired: 2 in, 2 out]
            n189 = property on="On/Off" class="Bool (strict)"("Visible"=w335, "Caption.Text"=w333) -> ()  [unwired: 2 in, 2 out]
          }
          frame "Compressor", "Digital Out" {
            w341 = FALSE ("Visible")
            # "Get direction and finish"
            n190 = property on="Motor" class="Clust (strict)"("Visible"=w341) -> ()  [unwired: 2 in, 2 out]
            n191 = property on="Test Slider" class="Slide (strict)"("Visible"=w341) -> ()  [unwired: 2 in, 2 out]
            n192 = property on="Test Ring" class="Ring (strict)"("Visible"=w341) -> ()  [unwired: 2 in, 2 out]
            n193 = property on="On/Off" class="Bool (strict)"("Visible"=TRUE, "Caption.Text"=w342) -> ()  [unwired: 2 in, 2 out]
            n194 = property on="Rev/Fwd" class="Clust (strict)"("Visible"=FALSE) -> ()  [unwired: 2 in, 2 out]
          }
          frame "Camera" {
            n195 = call <vilib>:"Get Last Path Segment.vi"("String in"=w349) -> ("String out"=w350:string)  [unwired: 10 in]
            n196 = property on="On/Off" class="Bool (strict)"("Visible"=FALSE) -> ()  [unwired: 2 in, 2 out]
            n197 = property on="Motor" class="Clust (strict)"("Visible"=FALSE) -> ()  [unwired: 2 in, 2 out]
            n198 = property on="Rev/Fwd" class="Clust (strict)"("Visible"=FALSE) -> ()  [unwired: 2 in, 2 out]
            n199 = case shown="\"White Balance  **\"" w350 {
              tunnel: w349 -> [w356 w365 w374 w383 w392 _ w398]
              tunnel: w348 -> [w354 w362 w371 w380 w389 _ _]
              frame "Size  **" {
                n200 = Index Array(array=w354) -> (element=w353:cluster{string[]})  [unwired: 1 in]
                n201 = call <vilib>:"NT Read String.vi"("Name"=w356) -> ("String"=w355:string)  [unwired: 9 in, 1 out]
                n202 = Unbundle(w353) -> (w351:string[])
                n203 = Match First String(2:w351, 3:w355) -> (0:w352:i32)  [unwired: 1 out]
                n204 = property on="Test Ring" class="Ring (strict)"("Value"=w352, "Strings []"=w351) -> ()  [unwired: 2 in, 2 out]
                n205 = property on="Test Ring" class="Ring (strict)"("Visible"=TRUE) -> ()  [unwired: 2 in, 2 out]
                n206 = property on="Test Slider" class="Slide (strict)"("Visible"=FALSE) -> ()  [unwired: 2 in, 2 out]
              }
              frame "White Balance  **" {
                n207 = Index Array(array=w362, index=1) -> (element=w363:cluster{string[]})
                n208 = call <vilib>:"NT Read String.vi"("Name"=w365) -> ("String"=w364:string)  [unwired: 9 in, 1 out]
                n209 = Unbundle(w363) -> (w360:string[])
                n210 = Match First String(2:w360, 3:w364) -> (0:w359:i32)  [unwired: 1 out]
                n211 = property on="Test Ring" class="Ring (strict)"("Value"=w359, "Strings []"=w360) -> ()  [unwired: 2 in, 2 out]
                n212 = property on="Test Ring" class="Ring (strict)"("Visible"=TRUE) -> ()  [unwired: 2 in, 2 out]
                n213 = property on="Test Slider" class="Slide (strict)"("Visible"=FALSE) -> ()  [unwired: 2 in, 2 out]
              }
              frame "Exposure  **" {
                n214 = Index Array(array=w371, index=2) -> (element=w372:cluster{string[]})
                n215 = call <vilib>:"NT Read String.vi"("Name"=w374) -> ("String"=w373:string)  [unwired: 9 in, 1 out]
                n216 = Unbundle(w372) -> (w368:string[])
                n217 = Match First String(2:w368, 3:w373) -> (0:w369:i32)  [unwired: 1 out]
                n218 = property on="Test Ring" class="Ring (strict)"("Value"=w369, "Strings []"=w368) -> ()  [unwired: 2 in, 2 out]
                n219 = property on="Test Ring" class="Ring (strict)"("Visible"=TRUE) -> ()  [unwired: 2 in, 2 out]
                n220 = property on="Test Slider" class="Slide (strict)"("Visible"=FALSE) -> ()  [unwired: 2 in, 2 out]
              }
              frame "Exposure Priority  **" {
                n221 = Index Array(array=w380, index=3) -> (element=w381:cluster{string[]})
                n222 = call <vilib>:"NT Read String.vi"("Name"=w383) -> ("String"=w382:string)  [unwired: 9 in, 1 out]
                n223 = Unbundle(w381) -> (w377:string[])
                n224 = Match First String(2:w377, 3:w382) -> (0:w378:i32)  [unwired: 1 out]
                n225 = property on="Test Ring" class="Ring (strict)"("Value"=w378, "Strings []"=w377) -> ()  [unwired: 2 in, 2 out]
                n226 = property on="Test Ring" class="Ring (strict)"("Visible"=TRUE) -> ()  [unwired: 2 in, 2 out]
                n227 = property on="Test Slider" class="Slide (strict)"("Visible"=FALSE) -> ()  [unwired: 2 in, 2 out]
              }
              frame "Color Enable  **" {
                n228 = Index Array(array=w389, index=4) -> (element=w390:cluster{string[]})
                n229 = call <vilib>:"NT Read String.vi"("Name"=w392) -> ("String"=w391:string)  [unwired: 9 in, 1 out]
                n230 = Unbundle(w390) -> (w386:string[])
                n231 = Match First String(2:w386, 3:w391) -> (0:w387:i32)  [unwired: 1 out]
                n232 = property on="Test Ring" class="Ring (strict)"("Value"=w387, "Strings []"=w386) -> ()  [unwired: 2 in, 2 out]
                n233 = property on="Test Ring" class="Ring (strict)"("Visible"=TRUE) -> ()  [unwired: 2 in, 2 out]
                n234 = property on="Test Slider" class="Slide (strict)"("Visible"=FALSE) -> ()  [unwired: 2 in, 2 out]
              }
              frame Default {
                n235 = property on="Test Ring" class="Ring (strict)"("Visible"=FALSE) -> ()  [unwired: 2 in, 2 out]
                n236 = property on="Test Slider" class="Slide (strict)"("Visible"=FALSE) -> ()  [unwired: 2 in, 2 out]
              }
              frame "Brightness  **", "Color Level  **", "Compression  **", "FPS  **", "Sharpness  **" {
                n237 = call <vilib>:"NT Read Number.vi"("Name"=w398) -> ("Numeric"=w397:dbl)  [unwired: 9 in, 1 out]
                n238 = local write "Test Slider"(w397) -> ()
                n239 = property on="Test Slider" class="Slide (strict)"("Visible"=TRUE, "Scale.Maximum"=100.0 ("Scale.Range:Maximum")) -> ()  [unwired: 2 in, 2 out]
                n240 = property on="Test Ring" class="Ring (strict)"("Visible"=FALSE) -> ()  [unwired: 2 in, 2 out]
              }
            }
          }
        }
        n241 = property on="Progress" class="Clust (strict)"("Visible"=FALSE) -> ()  [unwired: 2 in, 2 out]
      }
      event "Test Name": Mouse Enter {
        # "Populate the ring with the list of tests"
        n242 = event-data() -> ()  [unwired: 1 in, 1 out]
        n243 = call <vilib>:"NT Read String Array.vi"("Name"="TestMode/TestList") -> ("String Array"=w406:string[])  [unwired: 9 in, 1 out]
        n244 = Build Array (concatenate)("Select the test to run...", w406) -> (w405:string[])
        n245 = property on="Test Name" class="Ring (strict)"("Strings []"=w405) -> ()  [unwired: 2 in, 2 out]
      }
      event "Test Name": Value Change {
        w408 = FALSE ("Visible")
        # "Tell the robot the test name to run"
        n246 = event-data() -> ("NewVal"=w412:u16)  [unwired: 1 in]
        n247 = property on="Test Name" class="Ring (strict)"() -> ("Strings []"=w413:string[])  [unwired: 2 in, 2 out]
        n248 = local write "Progress"(T6 {"Test Progress"=0, "Test Progress Text"=""} ("Progress")) -> ()
        n249 = Index Array(array=w413, index=w412) -> (element=w411:string)
        n250 = call <vilib>:"NT Write String.vi"("String"=w411, "Name"="TestMode/TestName") -> ()  [unwired: 9 in, 1 out]
        n251 = property on="Progress" class="Clust (strict)"("Visible"=TRUE) -> ()  [unwired: 2 in, 2 out]
        n252 = property on="Motor" class="Clust (strict)"("Visible"=w408) -> ()  [unwired: 2 in, 2 out]
        n253 = property on="Test Slider" class="Slide (strict)"("Visible"=w408) -> ()  [unwired: 2 in, 2 out]
        n254 = property on="On/Off" class="Bool (strict)"("Visible"=w408) -> ()  [unwired: 2 in, 2 out]
        n255 = property on="Rev/Fwd" class="Clust (strict)"("Visible"=w408) -> ()  [unwired: 2 in, 2 out]
        n256 = property on="Test Ring" class="Ring (strict)"("Visible"=w408) -> ()  [unwired: 2 in, 2 out]
      }
      event "Select Auto": Mouse Enter {
        # "Populate the combo box with the list of autonomous options"
        n257 = event-data() -> ()  [unwired: 1 in, 1 out]
        n258 = call <vilib>:"NT Read String Array.vi"("Name"="Auto List") -> ("String Array"=w415:string[])  [unwired: 9 in, 1 out]
        n259 = property on="Select Auto" class="CmbBox"("Strings[]"=w415) -> ()  [unwired: 2 in, 2 out]
      }
      event "Select Auto": Value Change {
        # "User modified the Auto Selection. Write to NT variable so robot knows."
        n260 = event-data() -> ("NewVal"=w418:string)  [unwired: 1 in]
        n261 = call <vilib>:"NT Write String.vi"("String"=w418, "Name"="Auto Selector") -> ()  [unwired: 9 in, 1 out]
      }
      event "Command Selection": Value Change {
        # "Get the params and show in table"
        n262 = event-data() -> ("NewVal"=w424:i32)  [unwired: 1 in]
        n263 = property on="Command Selection" class="MCListbox (strict)"() -> ("ItemNames"=w422:string[][])  [unwired: 2 in, 2 out]
        n264 = call <vilib>:"WPI_DashboardUpdate Command Params.vi"("NewVal"=w424, "Commands"=w422, "Param Tbl"=w423) -> ()  [unwired: 8 in, 1 out]
      }
      event "Execute Command": Value Change {
        # "Started one, Unique ID holds\nresponse"
        n265 = event-data() -> ()  [unwired: 1 in, 1 out]
        n266 = property on="Command Selection" class="MCListbox (strict)"() -> ("ItemNames"=w435:string[][])  [unwired: 2 in, 2 out]
        n267 = Index Array(array=w435, index (row)="Command Selection", index (col)=0) -> (element=w433:string)
        n268 = call <vilib>:"Invoke Commands.vi"("Command Params"="Command Params", "Function Name"=w433) -> ("Params"=w429:u8, "Started"=w428:bool)  [unwired: 7 in, 1 out]
        n269 = Array Subset(array="Command Params", length (row)=w429) -> (w430:string[][])  [unwired: 3 in]
        n270 = Select(t="Executing" ("Cmd Status"), s=w428, f="" ("Cmd Status")) -> (s? t:f=→"Cmd Status":string)
      }
      event "Command Selection": Double Click {
        n271 = event-data() -> ("Row"=w443:i32)  [unwired: 1 in]
        n272 = property on="Command Selection" class="MCListbox (strict)"() -> ("ItemNames"=w446:string[][])  [unwired: 2 in, 2 out]
        n273 = local read "Command Params"() -> (w442:string[][])
        n274 = Index Array(array=w446, index (row)=w443, index (col)=0) -> (element=w444:string)
        n275 = call <vilib>:"Invoke Commands.vi"("Command Params"=w442, "Function Name"=w444) -> ("Params"=w441:u8, "Started"=w436:bool)  [unwired: 7 in, 1 out]
        n276 = Array Subset(array=w442, length (row)=w441) -> (w440:string[][])  [unwired: 3 in]
        n277 = Select(t="Executing" ("Cmd Status"), s=w436, f="" ("Cmd Status")) -> (s? t:f=w437:string)
        n278 = local write "Cmd Status"(w437) -> ()
      }
      event "CheckList": Double Click {
        # "Shift clears all"
        # "Update symbols on the listbox"
        n279 = event-data() -> ("PlatMods.Shift"=w448:bool, "Row"=w450:i32)  [unwired: 1 in]
        n280 = case shown="True" w448 {
          tunnel: w450 -> [w454 _]
          tunnel: 1 -> [w453 _]
          frame False {
            n281 = property on="CheckList" class="LstBox (strict)"() -> ("Item Symbols"=w452:i32[])  [unwired: 2 in, 2 out]
            n282 = Replace Array Subset(array=w452, new element=w453, index=w454) -> (w451:i32[])
            n283 = property on="CheckList" class="LstBox (strict)"("Item Symbols"=w451) -> ()  [unwired: 2 in, 2 out]
          }
          frame True {
            w455 = 0 ("Top Row")
            n284 = property on="CheckList" class="LstBox (strict)"() -> ("Number of Rows"=w457:u32)  [unwired: 2 in, 2 out]
            n285 = Initialize Array(0, w457) -> (w456:i32[])
            n286 = property on="CheckList" class="LstBox (strict)"("Top Row"=w455, "Value"=w455, "Item Symbols"=w456) -> ()  [unwired: 2 in, 2 out]
          }
        }
      }
      event "CheckList": Key Down {
        # "Update symbols on the listbox\nLeft and right keys check and uncheck"
        n287 = event-data() -> ("VKey"=w461:T23)  [unwired: 1 in]
        n288 = case shown="\"Left\", \"Right\"" w461 {
          selector: w461 -> [w466 _]
          tunnel: eventvkey."Left" ("VKey") -> [w464 _]
          frame "Left", "Right" {
            n289 = Equal?(x=w464, y=w466) -> (x = y?=w465:bool)
            n290 = Select(t=0, s=w465, f=1) -> (s? t:f=w467:i32)
            n291 = property on="CheckList" class="LstBox (strict)"() -> ("Item Symbols"=w470:i32[])  [unwired: 2 in, 2 out]
            n292 = Replace Array Subset(array=w470, new element=w467, index="CheckList") -> (w469:i32[])
            n293 = property on="CheckList" class="LstBox (strict)"("Item Symbols"=w469) -> ()  [unwired: 2 in, 2 out]
          }
          frame Default {
          }
        }
      }
      event "Motor.Enable": Value Change {
        # "When the test mode otor enable helper is set, update that\ntree row item's value"
        n294 = event-data() -> ("NewVal"=w476:bool)  [unwired: 1 in]
        n295 = Unbundle("Motor") -> ("Value"=w475:dbl)  [unwired: 1 out]
        n296 = Select(t=w475, s=w476, f=0.0) -> (s? t:f=w473:dbl)
        n297 = call <vilib>:"NT Write Number.vi"("Numeric"=w473, "Name"=w472) -> ()  [unwired: 9 in, 1 out]
      }
      event "Test Slider": Value Change {
        # "When the test mode slider helper is set, update that\ntree row item's value"
        n298 = event-data() -> ("NewVal"=w479:dbl)  [unwired: 1 in]
        n299 = call <vilib>:"NT Write Number.vi"("Numeric"=w479, "Name"=w480) -> ()  [unwired: 9 in, 1 out]
      }
      event "On/Off": Value Change {
        # "When the test mode on/off helper value is set, update that\ntree row item's value"
        n300 = event-data() -> ("NewVal"=w484:bool)  [unwired: 1 in]
        n301 = Boolean To (0,1)(Boolean=w484) -> (0, 1=w483:i16)
        n302 = call <vilib>:"NT Write Number.vi"("Numeric"=w483, "Name"=w482) -> ()  [unwired: 9 in, 1 out]
      }
      event "Rev/Fwd": Value Change {
        # "When the test mode helper value for relays is set, update that\ntree row item's value"
        n303 = event-data() -> ("NewVal.Forward"=w492:bool, "NewVal.Reverse"=w491:bool)  [unwired: 1 in]
        n304 = Boolean To (0,1)(Boolean=w492) -> (0, 1=w488:i16)
        n305 = Boolean To (0,1)(Boolean=w491) -> (0, 1=w490:i16)
        n306 = Negate(x=w490) -> (-x=w489:i16)
        n307 = Add(x=w488, y=w489) -> (x+y=w487:i16)
        n308 = call <vilib>:"NT Write Number.vi"("Numeric"=w487, "Name"=w486) -> ()  [unwired: 9 in, 1 out]
      }
      event "Test Ring": Value Change {
        # "When a test mode helper value is selected from the ring,\nset the tree item's variable to the string value"
        n309 = event-data() -> ("NewVal"=w496:u16)  [unwired: 1 in]
        n310 = property on="Test Ring" class="Ring (strict)"() -> ("Strings []"=w497:string[])  [unwired: 2 in, 2 out]
        n311 = Index Array(array=w497, index=w496) -> (element=w495:string)
        n312 = call <vilib>:"NT Write String.vi"("String"=w495, "Name"=w494) -> ()  [unwired: 9 in, 1 out]
      }
      event "Rec Mode": Value Change {
        # "Update globals for recording mode and path to read log from.\nClear when logging and let NetworkTables set path for vision to\nuse."
        n313 = event-data() -> ("NewVal"=w508:enum32{"Stop", "Record", "Playback"})  [unwired: 1 in]
        n314 = global write "WPI_DashboardLogging Global.vi" "Logging Filename"(path "") -> ()
        n315 = global write "WPI_DashboardLogging Global.vi" "Recording"(w508) -> ()
        n316 = case shown="\"Playback\"" w508 {
          tunnel: w507 -> [_ w510 w519]
          tunnel: [_ _ w518] -> w505
          tunnel: [_ _ w517] -> _
          tunnel: w503 -> [_ _ w515]
          tunnel: cluster{i32, i32} {-250, 170} -> [_ _ w514]
          tunnel: [_ _ T24 {"Image Size"=TRUE, "Image Type"=TRUE, "Pixel Value"=TRUE, "ROI Information"=TRUE, "Zoom Factor"=FALSE} ("Image Information Shown:All Elements")] -> w498
          tunnel: [_ _ TRUE ("Zoom Factor")] -> w499
          tunnel: w501 -> [_ _ w511]
          frame Default {
          }
          frame "Stop", "Record" {
            # "Place Window too"
            n317 = invoke class="VI" method="FP.Close"(reference=w510) -> (reference out=w509:refnum<vi>)  [unwired: 2 in, 2 out]
            n318 = invoke class="VI" method="Abort VI"(reference=w509) -> ()  [unwired: 2 in, 3 out]
          }
          frame "Playback" {
            n319 = call "Open Playback Panel.vi"("Offset"=w514, "DB VI Ref"=w515, "Playback in"=w519) -> ("Playback out"=w516:refnum<vi>)  [unwired: 8 in]
            n320 = register-events(w516, w511) -> (reference out=w518:refnum<event-registration>, error out=w517:errorcluster)  [unwired: 2 in]
          }
        }
        n321 = property on="Camera Image Right" class="ImageControl"("Image Information Shown"=w498, "Image Information Visible"=w499) -> ()  [unwired: 2 in, 2 out]
        n322 = property on="Camera Image" class="ImageControl"("Image Information Shown"=w498, "Image Information Visible"=w499) -> ()  [unwired: 2 in, 2 out]
        n323 = call <vilib>:"WPI_DashboardNT Log FieldName Cache.vi"("Operation"=enum16{"Lookup/Add", "Index", "Clear"}."Clear") -> ()  [unwired: 8 in, 3 out]
      }
      event Panel Close {
        w521 = enum32{"Stop", "Record", "Playback"}."Stop" ("Rec Mode")
        # "Playback window has been closed, abort"
        n324 = event-data() -> ()  [unwired: 1 in, 4 out]
        n325 = local write "Rec Mode"(w521) -> ()
        n326 = global write "WPI_DashboardLogging Global.vi" "Recording"(w521) -> ()
      }
      event Panel Close {
        # "Abort playback window and ourself"
        n327 = event-data() -> ()  [unwired: 1 in, 4 out]
        n328 = invoke class="VI" method="FP.Close"(reference=w525) -> (reference out=w524:refnum<vi>)  [unwired: 2 in, 2 out]
        n329 = invoke class="VI" method="Abort VI"(reference=w524) -> (error out=w523:errorcluster)  [unwired: 2 in, 2 out]
        n330 = invoke class="VI" method="Abort VI"(error in=w523) -> ()  [unwired: 2 in, 3 out]
      }
      event User Event {
        n331 = event-data() -> ("IDs"=w532:cluster{"RPC field ID":u16, "Unique ID":u16}, "String"=w531:string)  [unwired: 1 in]
        n332 = Bundle("IDs"=w532, "String"=w531) -> (w530:T10)  [unwired: 1 in]
        n333 = call <vilib>:"Retrieve RPC Response.vi"("RPC Response"=w530) -> ("Output"=w528:string[][])  [unwired: 10 in]
        n334 = Build Array (concatenate)(w526, w528) -> (w527:string[][])
        n335 = local write "Command Params"(w527) -> ()
        n336 = local write "Cmd Status"("" ("Cmd Status")) -> ()
      }
      event "Tree": Double Click {
        n337 = event-data() -> ("PlatMods"=w538:T27, "Tag"=w535:string)  [unwired: 1 in]
        n338 = Unbundle(w538) -> ("Shift"=w537:bool)  [unwired: 4 out]
        n339 = String Subset(string=w535, length (rest)=1 ("length (rest)")) -> (substring=w534:string)  [unwired: 1 in]
        n340 = Not(x=w537) -> (.not. x?=w536:bool)
        n341 = case shown="\"/\"" w534 {
          tunnel: w535 -> [_ w541]
          tunnel: w536 -> [_ w540]
          frame Default {
          }
          frame "/" {
            n342 = call <vilib>:"NT Update Persistence.vi"("Persistence"=w540, "Name"=w541) -> ()  [unwired: 9 in, 1 out]
          }
        }
      }
    }
  }
  n343 = local write "Dashboard Tab"(T2."Drive" ("Dashboard Tab")) -> ()
  n344 = property on="On/Off" class="Bool (strict)"("Visible"=w36) -> ()  [unwired: 2 in, 2 out]
  n345 = property on="Motor" class="Clust (strict)"("Visible"=w36) -> ()  [unwired: 2 in, 2 out]
  n346 = property on="Progress" class="Clust (strict)"("Visible"=w36) -> ()  [unwired: 2 in, 2 out]
  n347 = property on="Test Ring" class="Ring (strict)"("Visible"=w36) -> ()  [unwired: 2 in, 2 out]
  n348 = property on="Rev/Fwd" class="Clust (strict)"("Visible"=w36) -> ()  [unwired: 2 in, 2 out]
  n349 = while {
    tunnel: u16 1741 ("timeout ms (25000)") -> [w543]
    stop <- FALSE stop-if-true
    n350 = TCP Create Listener(10:w543) -> (0:w542:errorcluster, 3:w544:refnum<k5>)  [unwired: 4 in, 1 out]
    n351 = case shown="No Error" w542 {
      selector: w542 -> [w546 _]
      tunnel: w544 -> [w547 _]
      frame No Error {
        n352 = while {
          tunnel: w547 -> [w550]
          tunnel: w546 -> [w549]
          stop <- FALSE stop-if-true
          n353 = TCP Wait On Listener(8:w549, 11:w550) -> (0:w551:errorcluster, 4:w552:refnum<k5>)  [unwired: 2 in, 3 out]
          n354 = local write "TCP"(w552) -> ()
          n355 = case shown="No Error" w551 {
            frame No Error {
            }
            frame Error {
              n356 = Wait (ms)(milliseconds to wait=u32 1000) -> ()  [unwired: 1 out]
            }
          }
        }
      }
      frame Error {
        n357 = Wait (ms)(milliseconds to wait=u32 1000) -> ()  [unwired: 1 out]
      }
    }
  }
  n358 = local write "Command Selection"(u16 0 ("milliseconds to wait")) -> ()
  n359 = local write "Command Params"(string[][] [] ("Command Params")) -> ()
  n360 = global write "WPI_DashboardLogging Global.vi" "Recording"(w59) -> ()
  n361 = local write "Rec Mode"(w59) -> ()
  n362 = call <vilib>:"NT Write String.vi"("String"="Select Auto", "Name"="Auto Selector") -> ()  [unwired: 9 in, 1 out]
